vi "list all functions.vi"(11 "user module configuration in":refnum<class "user tag bus module configuration.lvclass">) -> (2 "functions":string[](array[string]), 3 "user module configuration out":refnum<class "user tag bus module configuration.lvclass">)   [LabVIEW 2013, in "user tag bus module configuration.lvclass"]
uses:
  user tag bus module configuration.lvclass
  user tag bus module configuration.lvclass/user tag bus module configuration.ctl
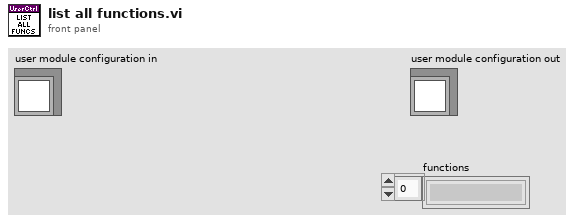
[diagram p1: front panel]
types:
  T1 = typedef "user tag bus module configuration.lvclass/control module configuration.ctl" = cluster{"name":string, "setpoint":refnum<class "TBM channel.lvclass">, "process variable":refnum<class "TBM channel.lvclass">, "output":refnum<class "TBM channel.lvclass">, "gains":T2, "output range":cluster{"output high":dbl, "output low":dbl}}
  T2 = typedef "user tag bus module configuration.lvclass/gains.ctl" = cluster{"Kp":dbl, "Ki":dbl, "Kd":dbl}
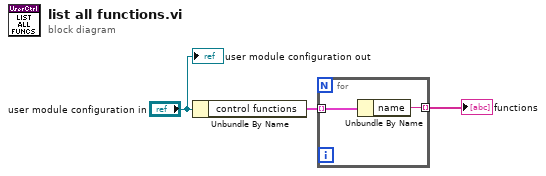
[diagram p0: block diagram]
diagram:
  n1 = Unbundle By Name("user module configuration in") -> ("control functions"=w2:T1[])
  n2 = for {
    tunnel: w2 -> [w5] mode=indexing
    tunnel: [w4] -> w1 mode=indexing
    n3 = Unbundle By Name(w5) -> ("name"=w4:string)
  }
  "functions" <- w1
  "user module configuration out" <- "user module configuration in"
